vi "nuke_database.vi"(8 "error IO 2":errorcluster) -> (0 "error IO":errorcluster, 3 "Database Nuked":bool)   [LabVIEW 2012]
uses:
  <vilib>/addons/database/NI_Database_API.lvlib
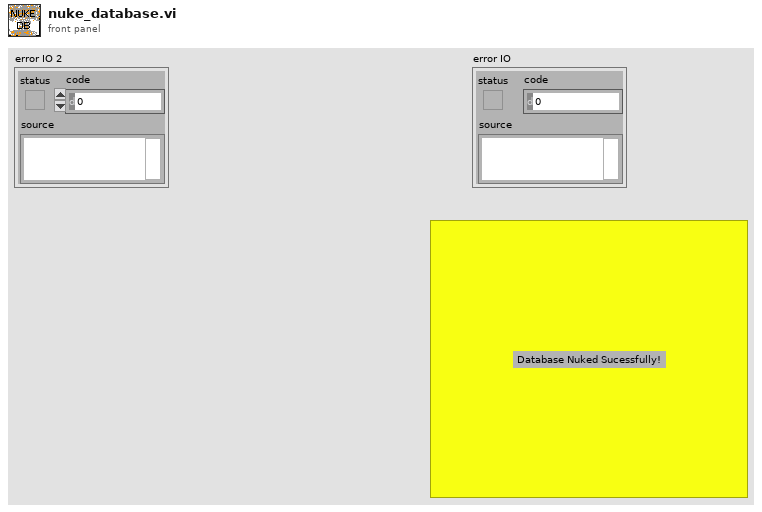
[diagram p1: front panel]
types:
  T1 = typedef "NI_Database_API.lvlib/Conn ObjectReference.ctl" = refnum<k1>
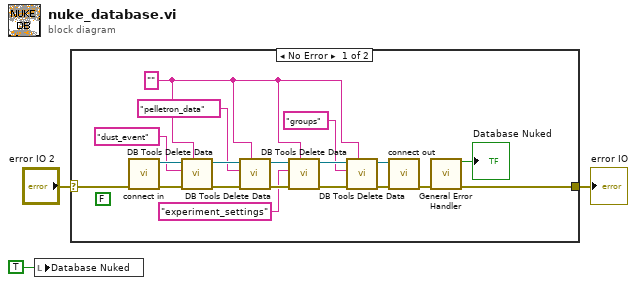
[diagram p0: block diagram]
diagram:
  n1 = local write "Database Nuked"(TRUE ("Database Nuked")) -> ()
  n2 = case shown="No Error" "error IO 2" {
    selector: "error IO 2" -> [w22 w23]
    tunnel: [w21 w23] -> w3
    frame No Error {
      w9 = "" ("condition")
      (unwired) FALSE
      n3 = call "connect in.vi"("error in (no error)"=w22) -> ("error out"=w16:errorcluster, "Database Connection"=w15:T1)  [unwired: 6 in, 1 out]
      n4 = call <vilib>:"DB Tools Delete Data.vi"("condition"=w9, "error in (no error)"=w16, "table"="dust_event", "connection reference"=w15) -> ("error out"=w18:errorcluster, "connection reference out"=w17:T1)  [unwired: 6 in]
      n5 = call <vilib>:"DB Tools Delete Data.vi"("condition"=w9, "error in (no error)"=w18, "table"="pelletron_data", "connection reference"=w17) -> ("error out"=w11:errorcluster, "connection reference out"=w12:T1)  [unwired: 6 in]
      n6 = call <vilib>:"DB Tools Delete Data.vi"("condition"=w9, "error in (no error)"=w11, "table"="experiment_settings", "connection reference"=w12) -> ("error out"=w8:errorcluster, "connection reference out"=w10:T1)  [unwired: 6 in]
      n7 = call <vilib>:"DB Tools Delete Data.vi"("condition"=w9, "error in (no error)"=w8, "table"="groups", "connection reference"=w10) -> ("error out"=w6:errorcluster, "connection reference out"=w7:T1)  [unwired: 6 in]
      n8 = call "connect out.vi"("error in (no error)"=w6, "connection reference"=w7) -> ("error out"=w19:errorcluster)  [unwired: 9 in]
      n9 = call <vilib>:"General Error Handler.vi"("error in (no error)"=w19) -> ("error?"=→"Database Nuked":bool, "error out"=w21:errorcluster)  [unwired: 10 in, 3 out]
    }
    frame Error {
    }
  }
  "error IO" <- w3
